vi "TestCloneAPI.vi"() -> ()   [LabVIEW 2014, in "SamplerModule.lvlib"]
uses:
  SamplerModule.lvlib
  SamplerPlugins/NISTSamplerPluginsBaseClass/TypeDefs/ConfigMeasurementParams.ctl
  SamplerPlugins/NISTSamplerPluginsBaseClass/TypeDefs/ConfigTriggerParams.ctl
  SamplerPlugins/NISTSamplerPluginsBaseClass/TypeDefs/ConfigACBandwidthParams.ctl
  SamplerPlugins/NISTSamplerPluginsBaseClass/TypeDefs/ConfigMultiPointParams.ctl
  SamplerPlugins/NISTSamplerPluginsBaseClass/TypeDefs/MultiPointReadingArrayParams.ctl
  SamplerPlugins/NISTSamplerPluginsBaseClass/TypeDefs/MultiPointReadingParams.ctl
  WfrmGenerator/WfrmPlugins/EventPluginBaseClass/TypeDefs/dblEvtSignalArray.ctl
  SamplerPlugins/NISTSamplerPluginsBaseClass/TypeDefs/CorrectionFactors.ctl
  <userlib>/NIST/ModuleAdminLib/ModuleAdmin/ModuleAdmin.lvclass
  PublicAPI/Arguments/Broadcasts/clDidInit.ctl
  <userlib>/NIST/ModuleAdminLib/ModuleAdmin/ModuleAdmin.lvclass/ModuleAdmin.ctl
  PublicAPI/Arguments/Requests/clStopArgument.ctl
  <userlib>/NIST/ModuleAdminLib/ModuleAdmin/Accessors/Read CloneRegRef.vi
  <userlib>/NIST/ModuleAdminLib/CloneRegistration/CloneRegistration.lvclass
  SamplerPlugins/NISTSamplerPluginsBaseClass/SamplerPluginsBase.lvclass
  SamplerPlugins/Simulation/Simulation.lvclass
  WfrmGenerator/WfrmPlugins/EventPluginBaseClass/BaseWfrmPlugin.lvclass
panel:
  in  "btnPref":bool
  in  "CorrectionFactors":T1
  in  "Plugin Type":u16(ring) items=["HP3458aDMM", "HIL Sampler", "NI Dyn3 Sampler", "NiPxi6123", "Sim"]
  in  "dblEventSignalArray":T2=array6x24000[144000 elements]
  in  "btnEvtSignal":bool
  in  "Loop Wait":u32=1000
  out "Waveform Chart":dbl[](graph)
  out "Stop":bool=TRUE
  out "Count":i32
  in  "btnLoopMultiPointReading":bool
  out "ReadingArray":dbl[](array[numeric])
  in  "btnInitiateMultiPoint":bool
  out "Waveform Graph":dbl[][](graph)
  out "MultiPointReadingArray":T3 {"Timestamp" format="%.6f"}
  in  "btnRequestMultiPointReading":bool
  in  "btnFetchMultiPoint":bool
  in  "btnReadMultiPoint":bool
  in  "ConfigMultiPointParams":T5={"iTriggerCount"=1, "iSampleCount"=4800, "eSampleClock"=2, "dSampleInterval"=0.00020833333333333332} {"eSampleClock" items=["NULL"=0, "Immediate"=1, "External"=2, "Software Trigger"=3, "Interval"=10]}
  in  "btnConfigMultiPoint":bool
  in  "eMeasCompleteDest":u16(ring) items=["None"=0, "External"=2]
  in  "btnConfigMeasCompDest":bool
  out "IsOverRange?":bool
  in  "dFrequencyVoltageRange":dbl
  in  "ConfigACBandwidthParams":T6
  in  "btnIsOverRange":bool
  in  "btnConfigACBandwidth":bool
  in  "btnConfigFreqVoltRange":bool
  in  "ConfigTriggerParams":T7={"eTriggerSource"=2, "dTriggerDelay"=0.0} {"eTriggerSource" items=["NULL", "Immediate", "External", "Software Trigger"]}
  in  "btnConfigTrigger":bool
  in  "btnInitiate":bool
  in  "iMaxTimeMillisecondsFetch":i32
  in  "btnFetch":bool
  in  "btnAbort":bool
  in  "btnReset":bool
  in  "btnInitializeDevice":bool
  in  "btnRequestReading":bool
  in  "iMaxTimeMilliseconds":i32
  in  "btnRead":bool
  in  "btnConfigMeasurement":bool
  in  "ConfigMeasurement":T8={"eFunction"=1, "dRange"=10.0, "dResolution"=0.0} {"eFunction" items=["NULL"=0, "DC Volts"=1, "AC Volts"=2, "DC Current"=3, "AC Current"=4, "Frequency"=104, "Period"=105, "AC Plus DC Volts"=106, "AC Plus DC Current"=107, "AC Coupled Direct Sampling"=1005, "DC Coupled Direct Sampling"=1006, "AC Coupled Sub Sampling"=1007, "DC Coupled Sub Sampling"=1008]}
  in  "btnLoadPlugin":bool
  out "Path":path
  in  "btnRequestINIPath":bool
  in  "btnRemove":bool
  out "Status Log":string
  out "Active Modules (Array)":string[](array[string])
  in  "btnAdd":bool
  in  "btnStop":bool
  in  "Select Module":i32(ring)=-1 caption="Select Module to send Request" items=["All"=-1]
  # "READING FROM .INI ONLY"
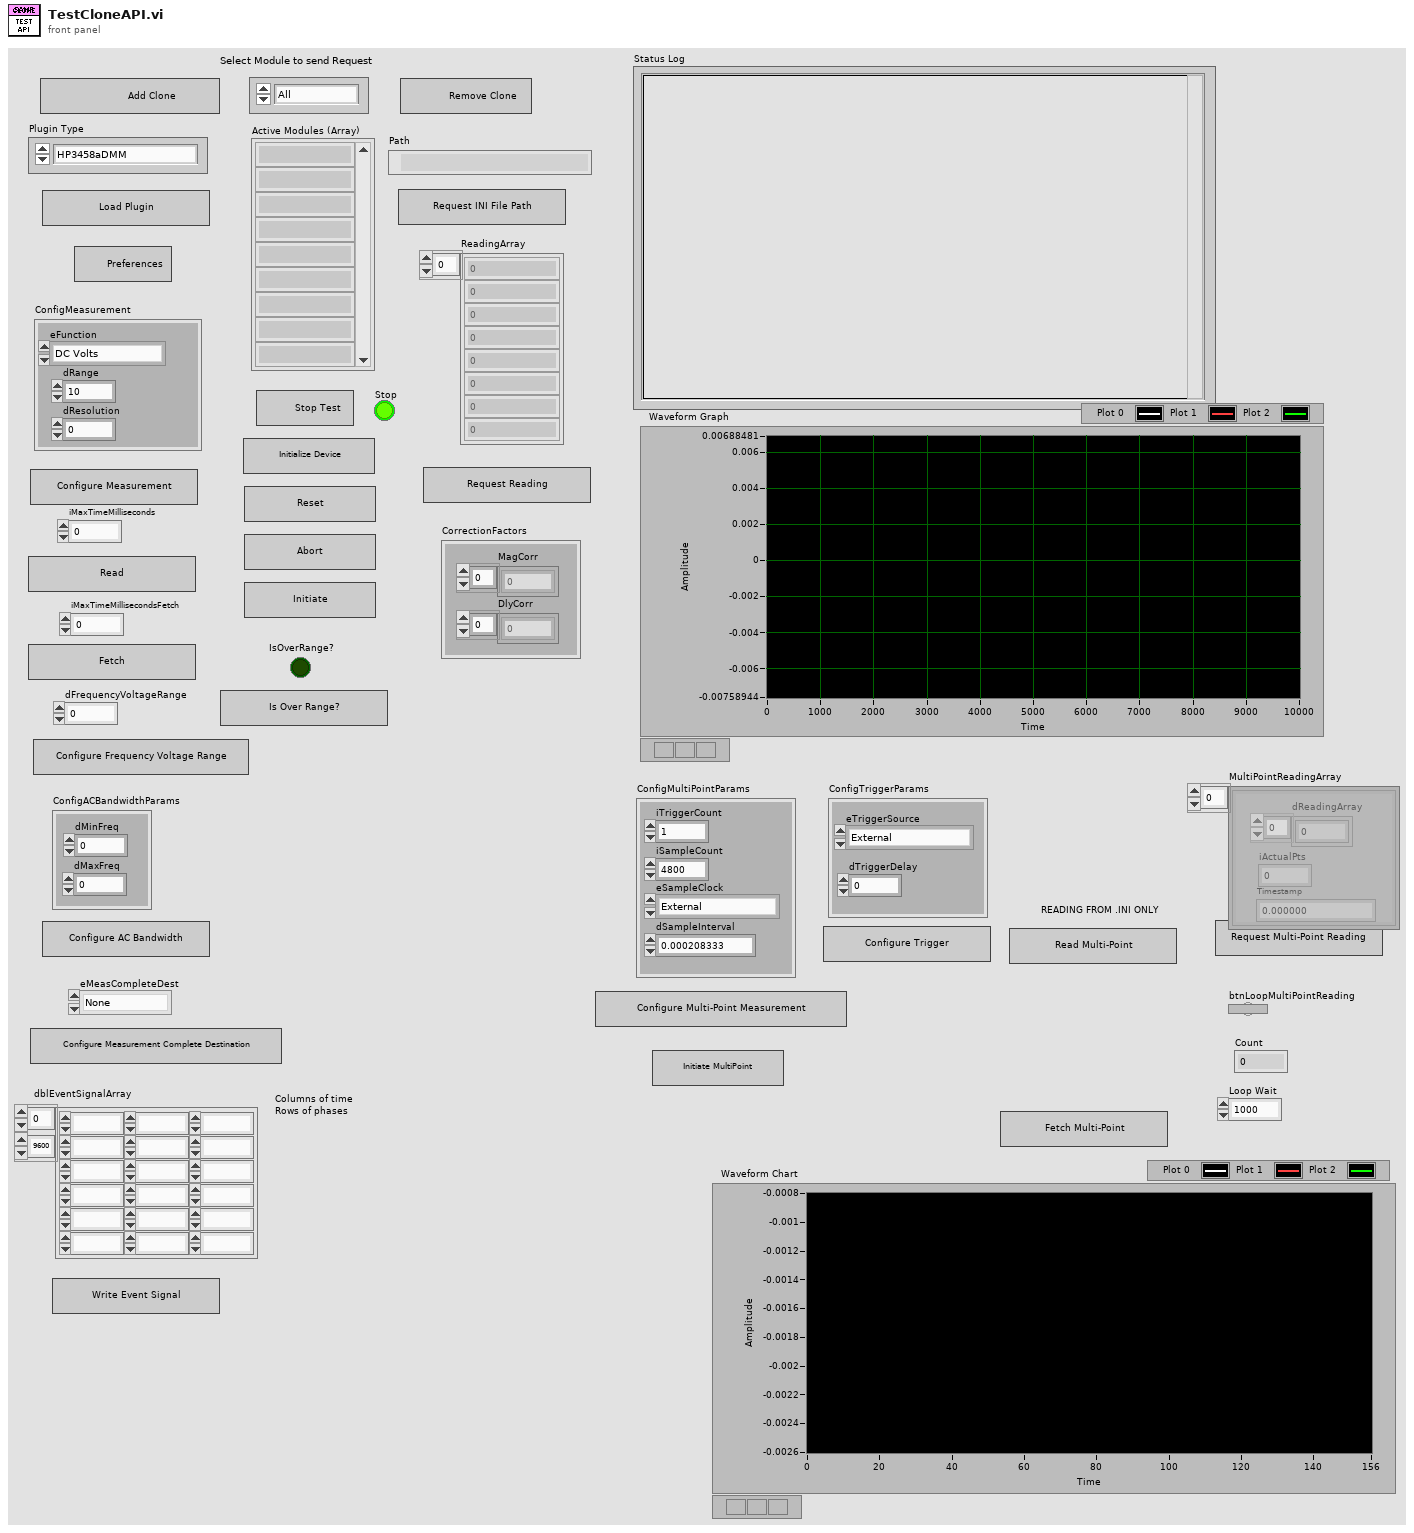
[diagram p1: front panel]
types:
  T1 = typedef "SamplerPlugins.lvlib/SamplerPluginsBase.lvclass/CorrectionFactors.ctl" = cluster{"MagCorr":dbl[], "DlyCorr":dbl[]}
  T2 = typedef "WfrmPlugins.lvlib/BaseWfrmPlugin.lvclass/dblEvtSignalArray.ctl" = dbl[][]
  T3 = typedef "SamplerPlugins.lvlib/SamplerPluginsBase.lvclass/MultiPointReadingArrayParams.ctl" = T4[]
  T4 = typedef "SamplerPlugins.lvlib/SamplerPluginsBase.lvclass/MultiPointReadingParams.ctl" = cluster{"dReadingArray":dbl[], "iActualPts":i32, "Timestamp":dbl}
  T5 = typedef "SamplerPlugins.lvlib/SamplerPluginsBase.lvclass/ConfigMultiPointParams.ctl" = cluster{"iTriggerCount":i32, "iSampleCount":i32, "eSampleClock":u16, "dSampleInterval":dbl}
  T6 = typedef "SamplerPlugins.lvlib/SamplerPluginsBase.lvclass/ConfigACBandwidthParams.ctl" = cluster{"dMinFreq":dbl, "dMaxFreq":dbl}
  T7 = typedef "SamplerPlugins.lvlib/SamplerPluginsBase.lvclass/ConfigTriggerParams.ctl" = cluster{"eTriggerSource":u16, "dTriggerDelay":dbl}
  T8 = typedef "SamplerPlugins.lvlib/SamplerPluginsBase.lvclass/ConfigMeasurementParams.ctl" = cluster{"eFunction":u16, "dRange":dbl, "dResolution":dbl}
  T9 = typedef "SamplerModule.lvlib/clBroadcastEvents.ctl" = cluster{"DidInit":refnum<user-event>, "StatusUpdate":refnum<user-event>, "ErrorReport":refnum<user-event>, "DidStop":refnum<user-event>, "PathToINI":refnum<user-event>, "GetReading":refnum<user-event>, "IsOverRange":refnum<user-event>, "GetMultiPointReading":refnum<user-event>, "MultiPointParams":refnum<user-event>, "MultiPointConfig":refnum<user-event>, "CorrFactors":refnum<user-event>}
  T10 = typedef "SamplerModule.lvlib/clDidInit.ctl" = cluster{"Init?":bool, "ModuleAdmin":refnum<class "ModuleAdmin.lvclass">}
  T11 = typedef "SamplerModule.lvlib/clStopArgument.ctl" = cluster{"Exit via Stop Module Req?":bool, "Wait for Module to stop?":bool, "ModuleAdmin":refnum<class "ModuleAdmin.lvclass">}
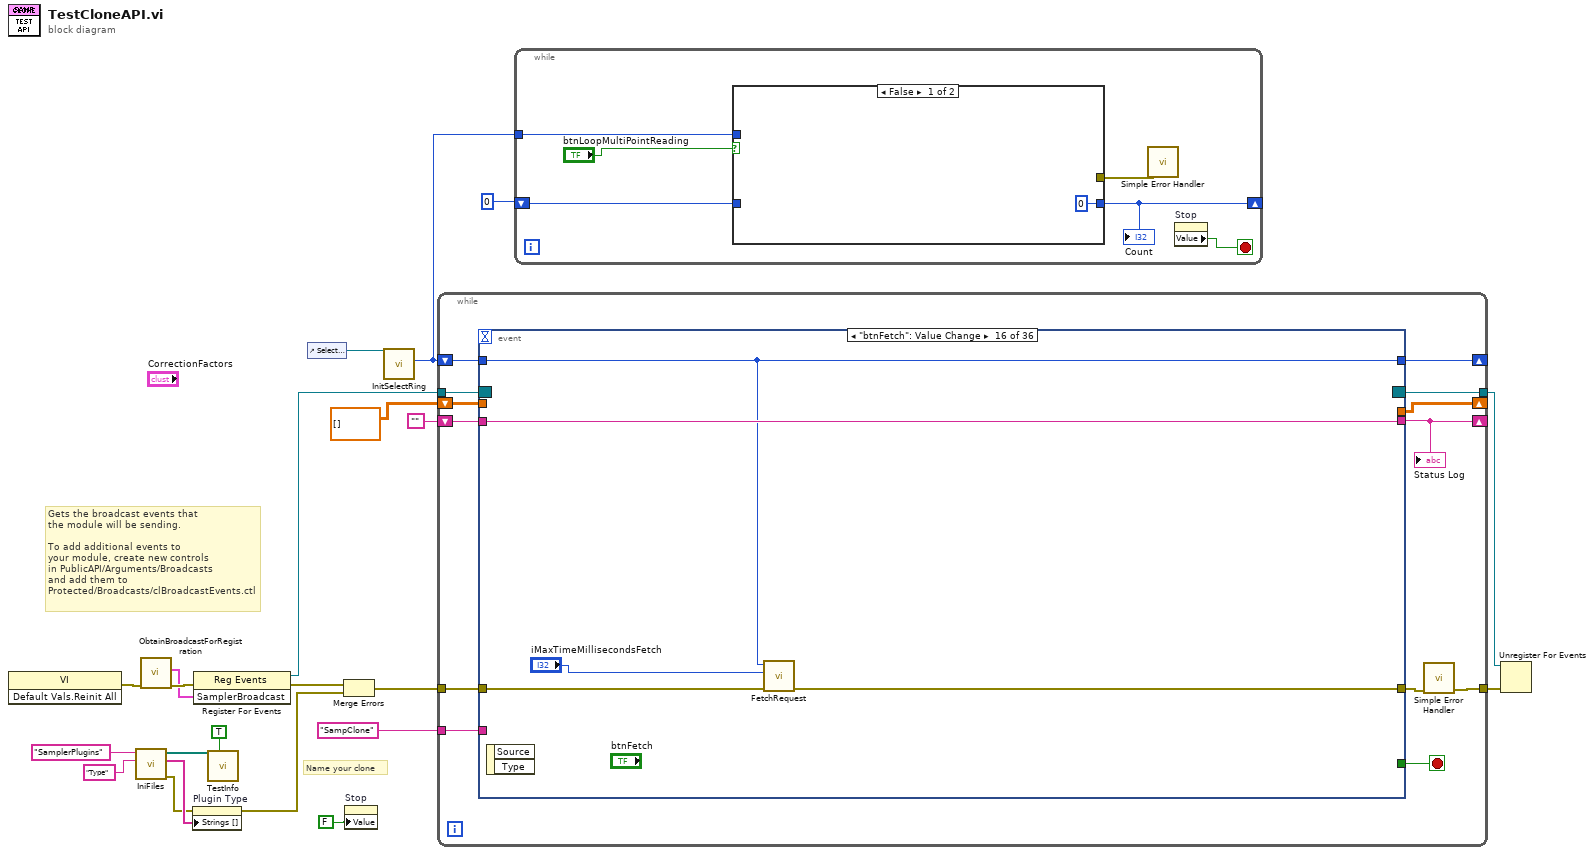
[diagram p0: block diagram]
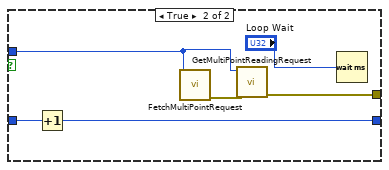
[diagram p2: hidden frame]
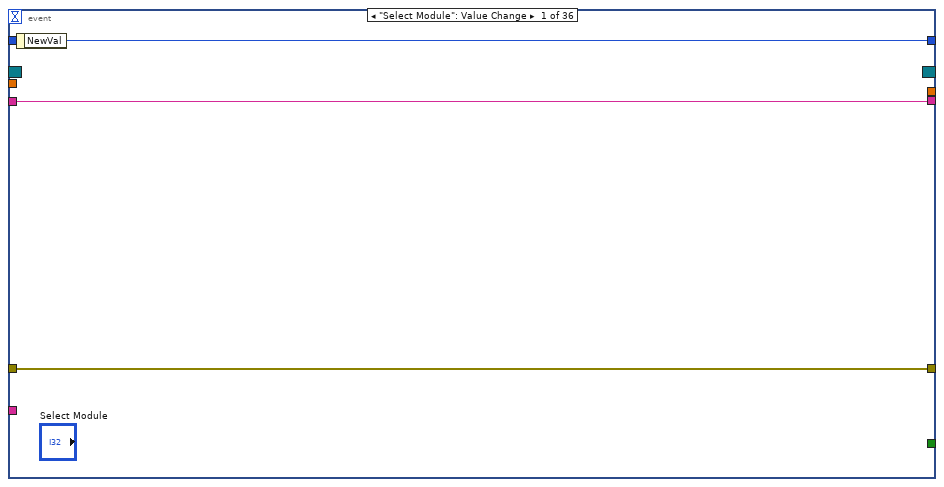
[diagram p3: hidden frame]
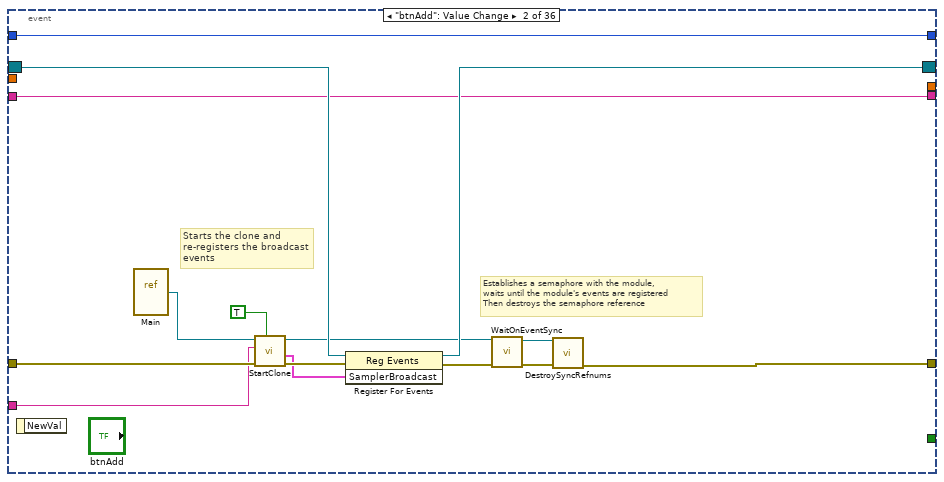
[diagram p4: hidden frame]
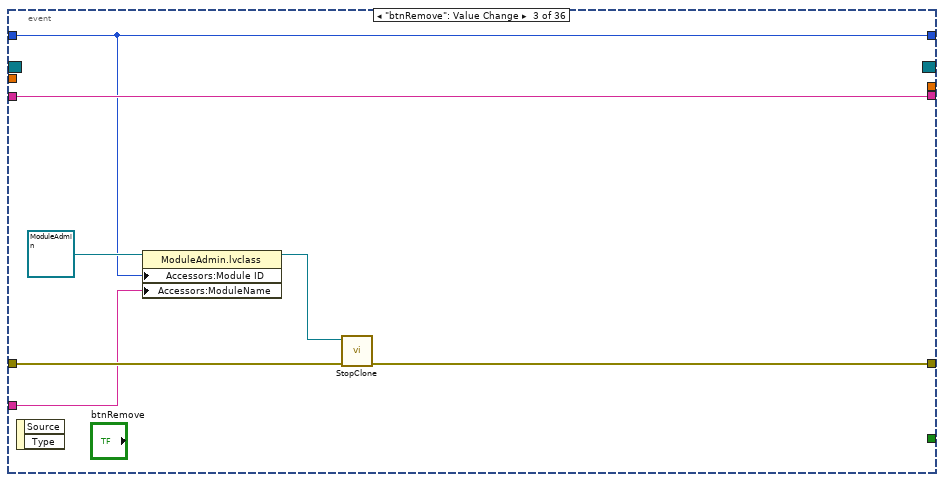
[diagram p5: hidden frame]
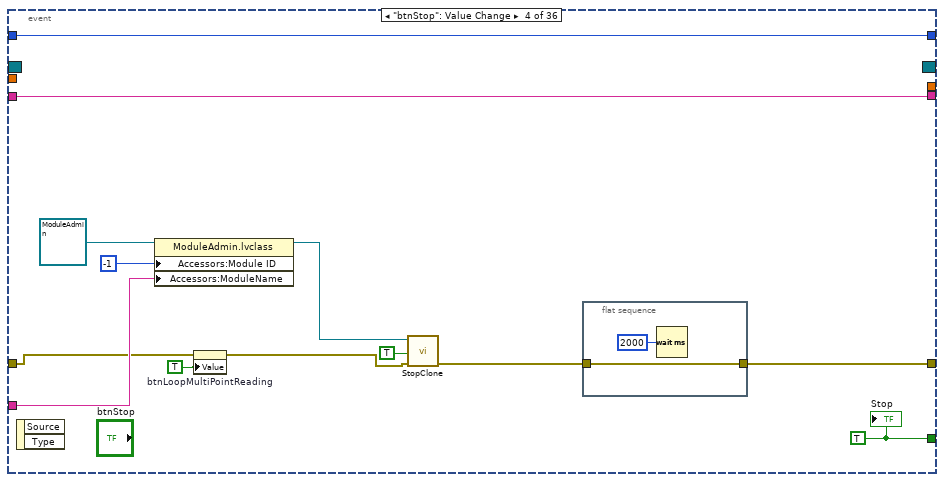
[diagram p6: hidden frame]
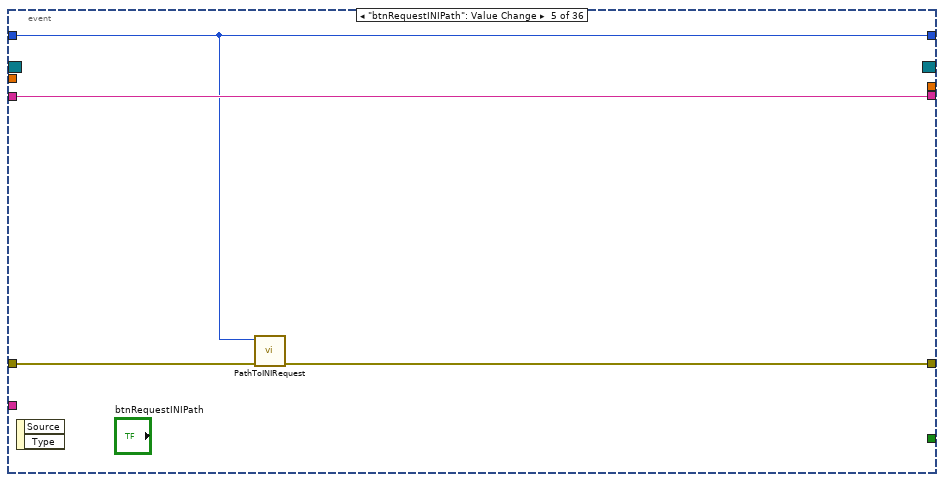
[diagram p7: hidden frame]
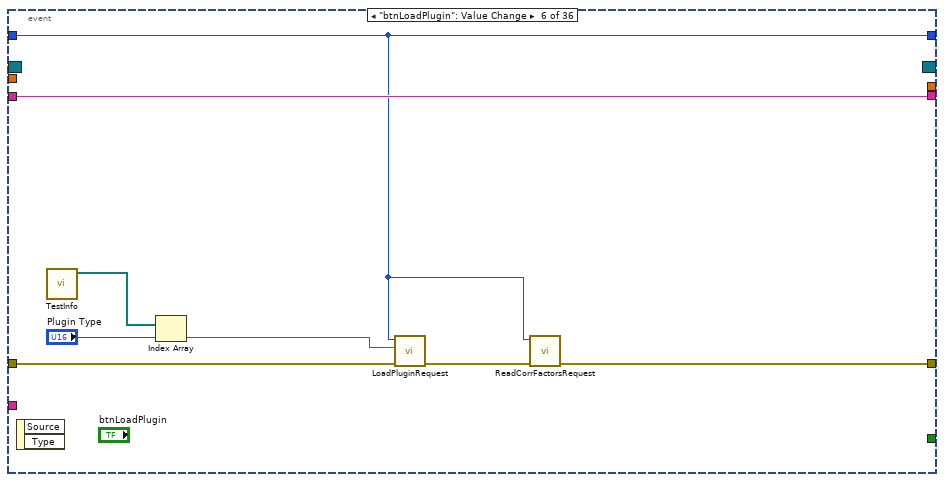
[diagram p8: hidden frame]
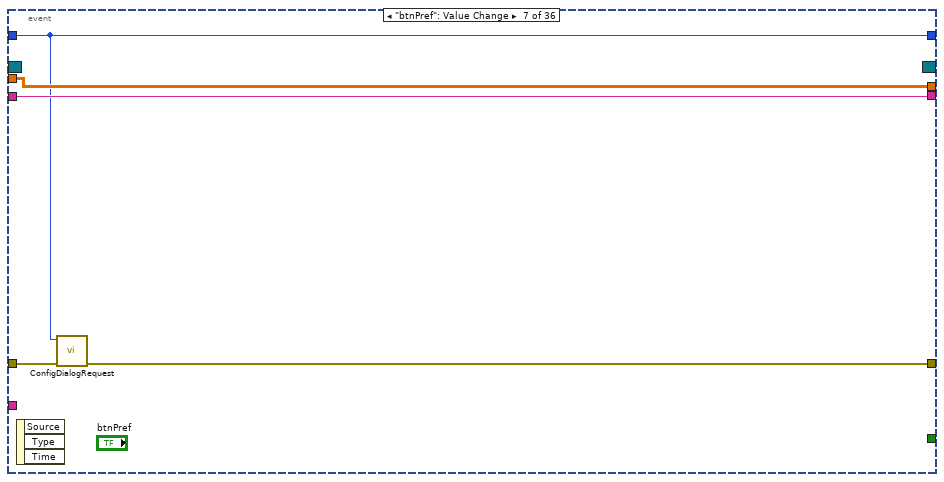
[diagram p9: hidden frame]
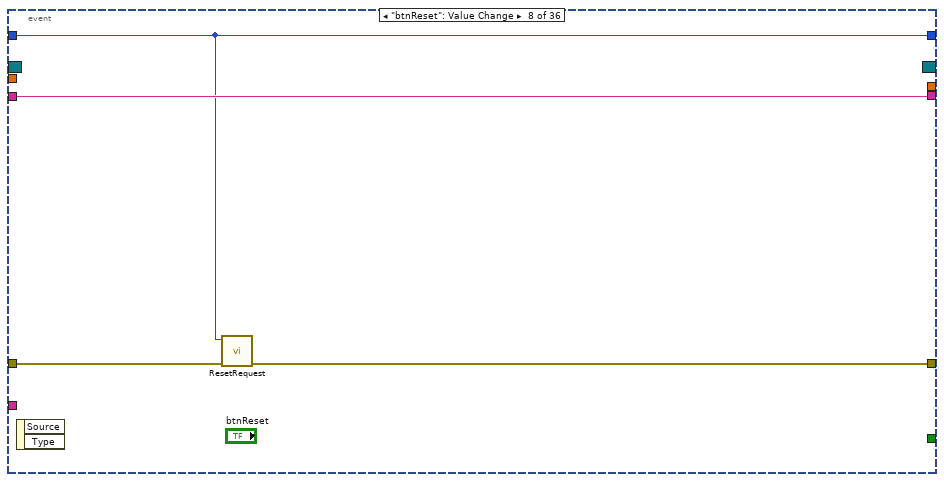
[diagram p10: hidden frame]
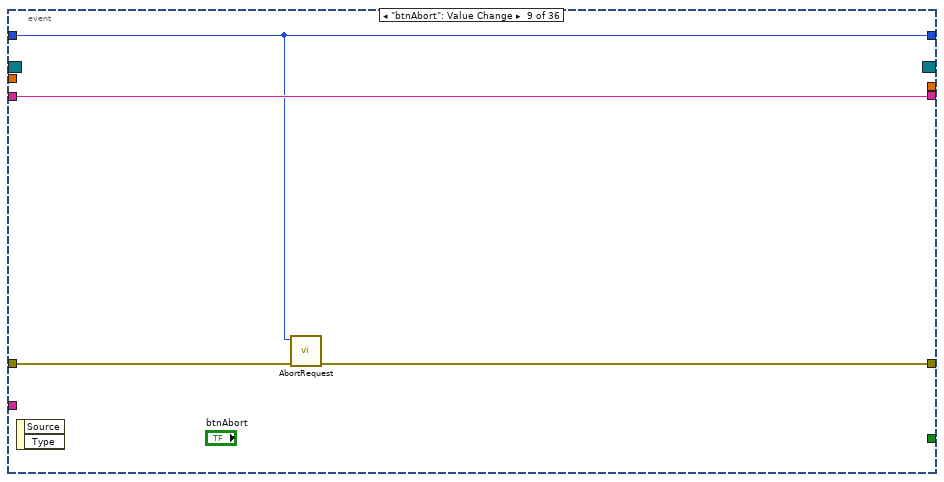
[diagram p11: hidden frame]
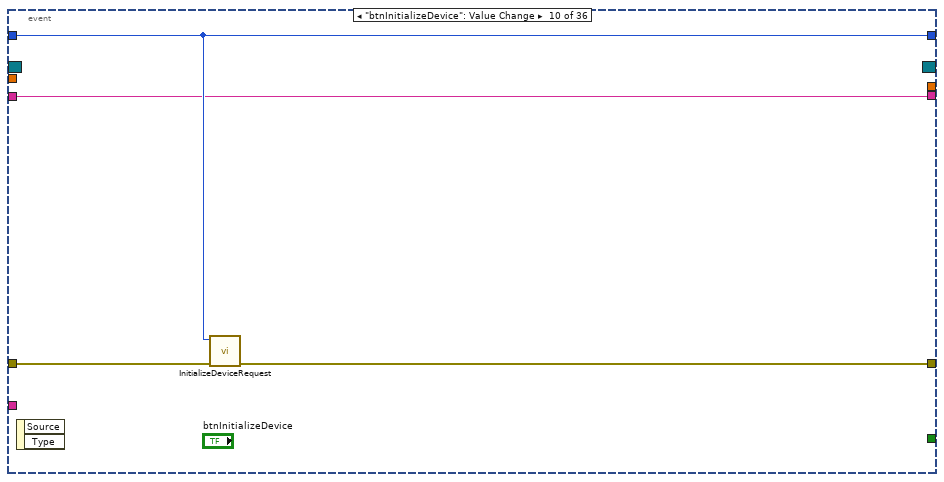
[diagram p12: hidden frame]
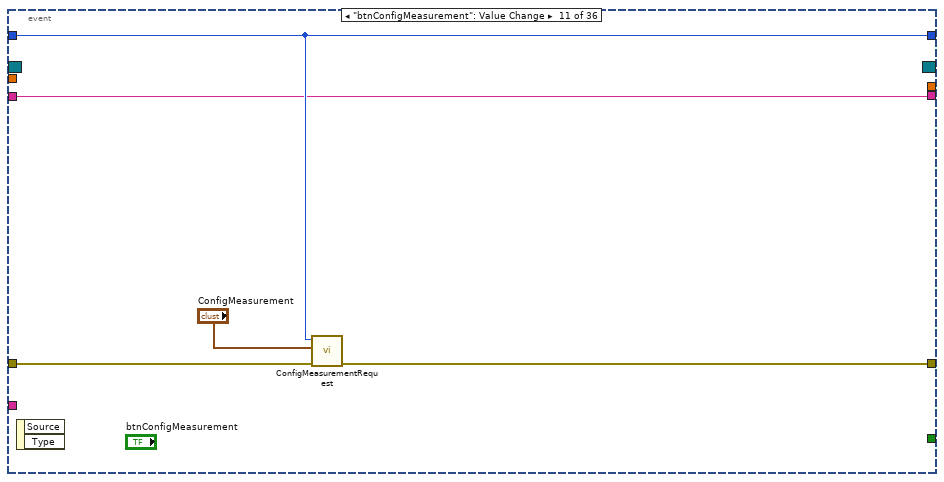
[diagram p13: hidden frame]
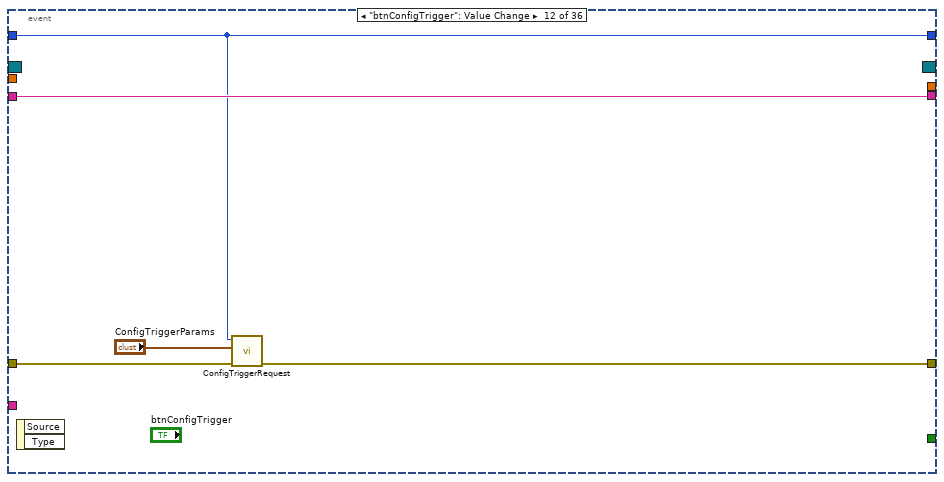
[diagram p14: hidden frame]
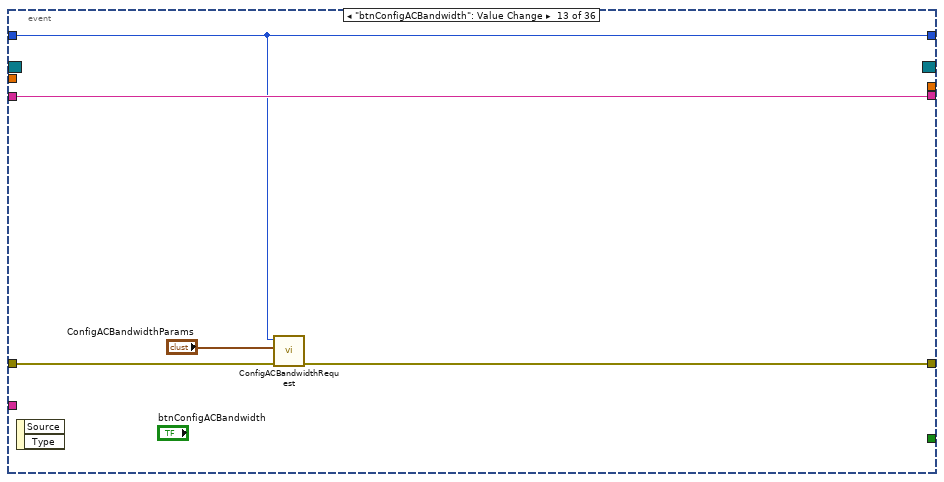
[diagram p15: hidden frame]
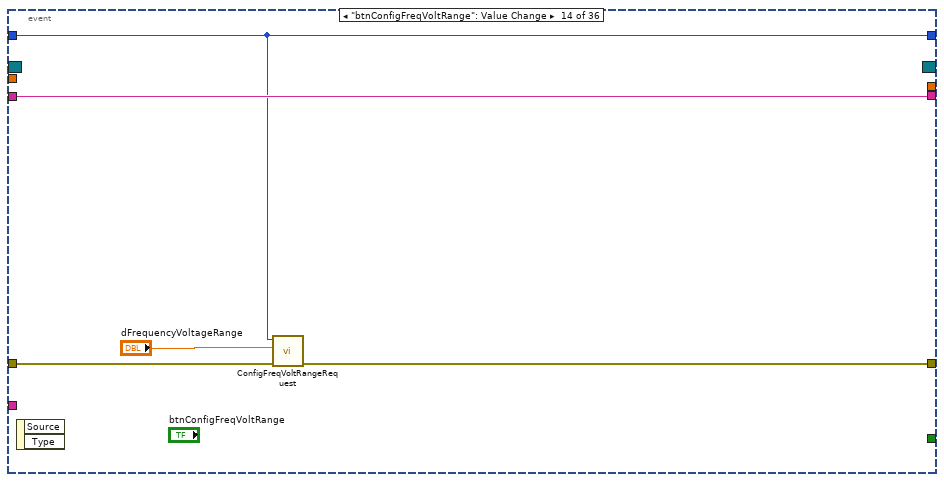
[diagram p16: hidden frame]
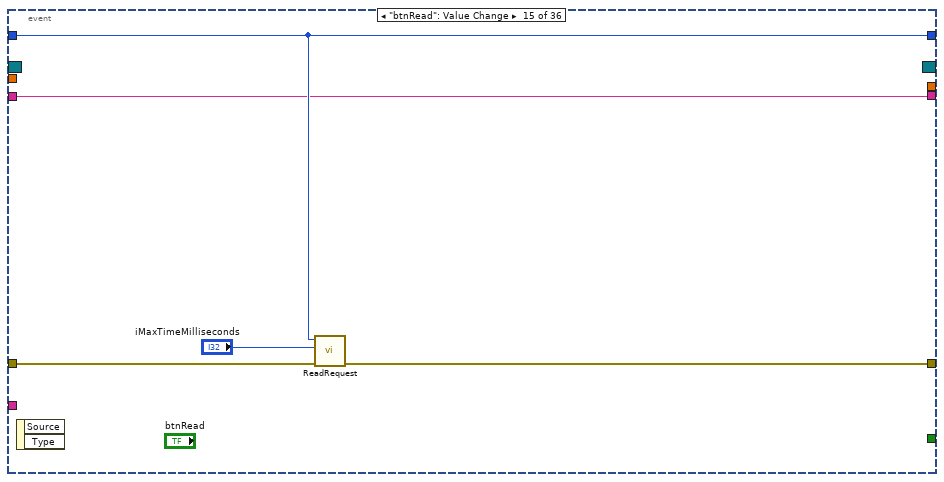
[diagram p17: hidden frame]
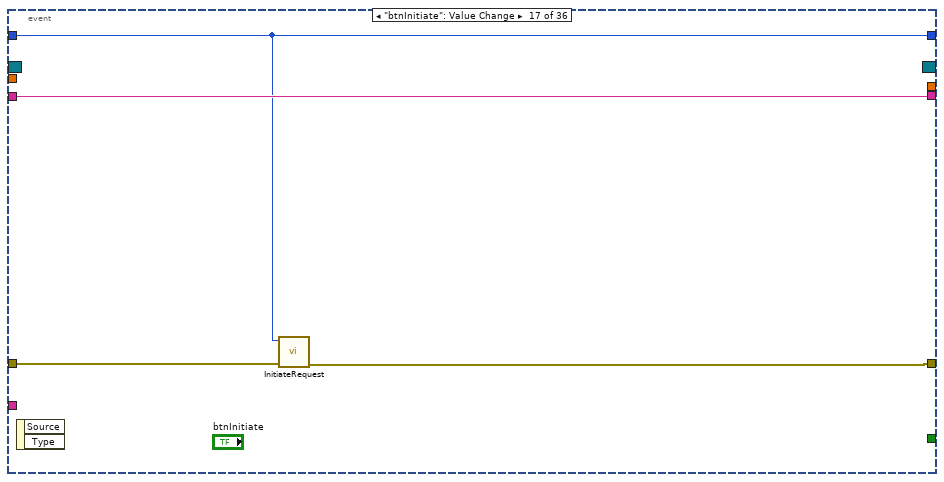
[diagram p18: hidden frame]
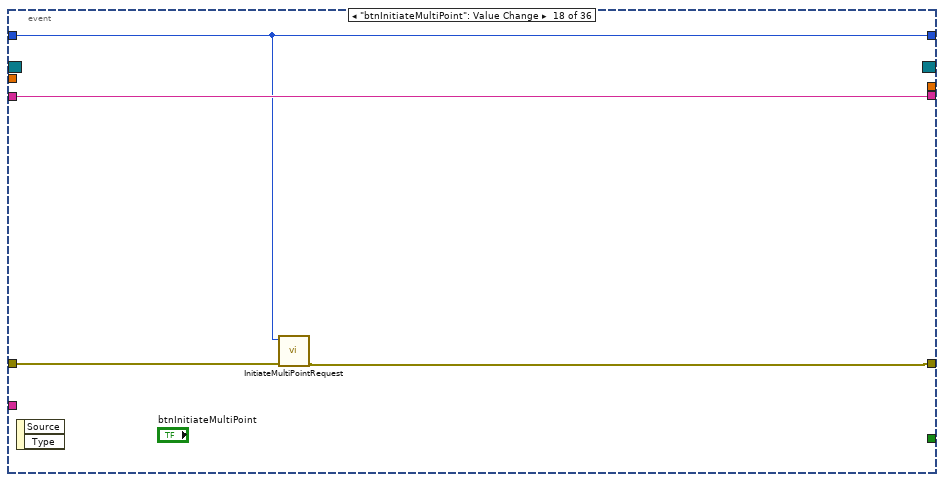
[diagram p19: hidden frame]
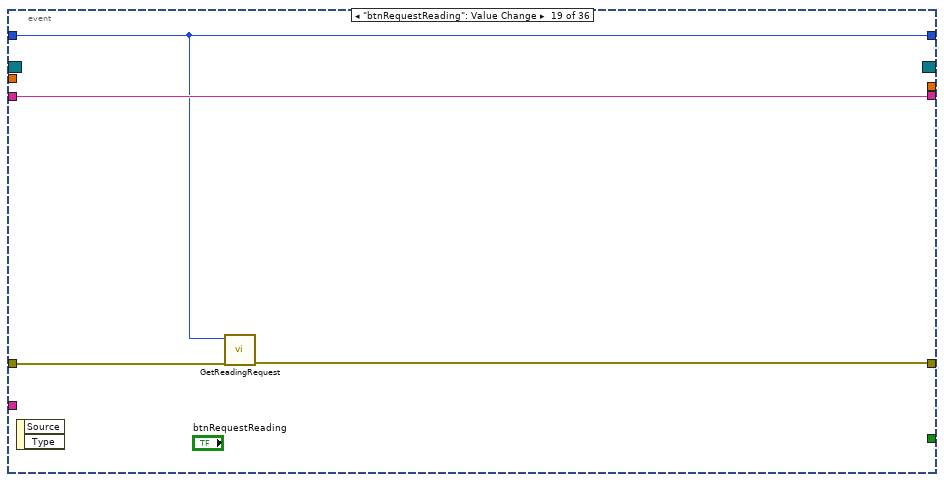
[diagram p20: hidden frame]
diagram:
  # "Name your clone"
  # "Gets the broadcast events that\nthe module will be sending.\n\nTo add additional events to\nyour module, create new controls\nin PublicAPI/Arguments/Broadcasts\nand add them to\nProtected/Broadcasts/clBroadcastEvents.ctl"
  n1 = invoke class="VI" method="Default Vals.Reinit All"() -> (error out=w21:errorcluster)  [unwired: 3 in, 2 out]
  n2 = call "IniFiles.vi"("iniKey"="Type", "name or relative path"="SamplerPlugins") -> ("error out"=w7:errorcluster, "Types"=w8:string[], "IniFilePaths"=w3:path[])  [unwired: 7 in]
  n3 = call "ObtainBroadcastForRegistration.vi"("error in (no error)"=w21) -> ("error out"=w20:errorcluster, "SamplerBroadcast"=w19:T9)  [unwired: 9 in]
  n4 = property on="Plugin Type" class="Ring (strict)"(error in=w7, "Strings []"=w8) -> (error out=w5:errorcluster)  [unwired: 1 in, 1 out]
  n5 = register-events(error in=w20, w19) -> (reference out=w17:refnum<event-registration>, error out=w18:errorcluster)  [unwired: 1 in]
  n6 = call "TestInfo.vi"("Set (f)"=TRUE, "PluginIniFilePaths"=w3) -> ()  [unwired: 9 in, 1 out]
  n7 = control-ref of="Select Module"() -> (w22:refnum<vi>)
  n8 = Merge Errors(w18, w5) -> (w6:errorcluster)
  n9 = property on="Stop" class="Bool (strict)"("Value"=FALSE ("Stop")) -> ()  [unwired: 2 in, 2 out]
  n10 = call "InitSelectRing.vi"("Ring Refnum"=w22) -> ("Module Ring Value"=w14:i32)  [unwired: 9 in, 1 out]
  n11 = while {
    shift-right: [w35] -> _
    shift-left: w14 -> [w26]
    tunnel: w6 -> [w33]
    tunnel: w17 -> [w30]
    tunnel: [w31] -> w2
    shift-right: [w29] -> _
    shift-left: "" -> [w28]
    tunnel: "SampClone" ("ModuleName") -> [w27]
    shift-right: [w24] -> _
    shift-left: dbl[][] [] -> [w25]
    tunnel: [w23] -> w1
    stop <- w34 stop-if-true
    n12 = event shown="[15] \"btnFetch\": Value Change" {
      selector: w30 -> [_ w45 _ _ _ _ _ _ _ _ _ _ _ _ _ _ _ _ _ _ _ _ _ _ _ _ _ _ _ _ _ _ _ _ _ _]
      dyn-events: [_ w44 _ _ _ _ _ _ _ _ _ _ _ _ _ _ _ _ _ _ _ _ _ _ _ _ _ _ _ _ _ _ _ _ _ _] -> w23
      timeout: _ -> [_ _ _ _ _ _ _ _ _ _ _ _ _ _ _ _ _ _ _ _ _ _ _ _ _ _ _ _ _ _ _ _ _ _ _ _]
      tunnel: w26 -> [_ w53 w56 w73 w78 w80 w89 w93 w97 w103 w109 w111 w115 w121 w129 w131 w137 w141 w143 w147 w151 w156 w161 w165 w169 w174 _ _ w243 w247 w258 w265 w272 w292 w301 w306]
      tunnel: [w38 w53 w56 w73 w78 w80 w89 w93 w97 w103 w109 w111 w115 w121 w129 w131 w137 w141 w143 w147 w151 w156 w161 w165 w169 w174 w200 w215 w243 w247 w258 w265 w272 w292 w301 w306] -> w35
      tunnel: [_ _ _ w72 _ _ _ _ _ _ _ _ _ _ _ _ _ _ _ _ _ _ _ _ _ _ _ _ _ _ _ _ _ _ _ _] -> w34
      tunnel: w33 -> [w36 w52 w59 w64 w77 w86 w92 w95 w99 w104 w107 w113 w118 w122 w127 w133 w136 w140 w145 w149 w155 w160 w164 w168 w172 w176 w205 w224 w240 w251 w254 w263 w270 w278 w299 w307]
      tunnel: [w36 w46 w58 w61 w76 w81 w88 w94 w98 w101 w106 w112 w117 w123 w126 w132 w135 w139 w144 w148 w154 w159 w163 w167 w171 w175 w189 w212 w234 w250 w253 w262 w269 w290 w294 w303] -> w32
      tunnel: [w37 w42 w60 w70 w79 w87 w91 w96 w100 w102 w105 w114 w119 w124 w125 w134 w138 w142 w146 w150 w152 w157 w162 w166 w170 w173 w193 w221 w237 w246 w259 w266 w273 w293 w300 w305] -> w29
      tunnel: w28 -> [w37 w42 w60 w70 w79 w87 w91 w96 w100 w102 w105 w114 w119 w124 w125 w134 w138 w142 w146 w150 w152 w157 w162 w166 w170 w173 w192 w222 w242 w246 w259 w266 w273 w293 w300 w305]
      tunnel: w27 -> [_ w41 w55 w67 _ _ _ _ _ _ _ _ _ _ _ _ _ _ _ _ _ _ _ _ _ _ _ _ _ _ _ _ _ _ _ _]
      tunnel: [_ _ _ _ _ _ w90 _ _ _ _ _ _ _ _ _ _ _ _ _ _ _ _ _ _ _ _ _ _ _ _ _ _ w275 _ w304] -> w24
      tunnel: w25 -> [_ _ _ _ _ _ w90 _ _ _ _ _ _ _ _ _ _ _ _ _ _ _ _ _ _ _ _ _ _ _ _ _ _ w276 _ w304]
      event "Select Module": Value Change {
        n13 = event-data() -> ("NewVal"=w38:i32)  [unwired: 1 in]
      }
      event "btnAdd": Value Change {
        # "Establishes a semaphore with the module,\nwaits until the module's events are registered\nThen destroys the semaphore reference"
        # "Starts the clone and\nre-registers the broadcast \nevents"
        n14 = event-data() -> ()  [unwired: 1 in, 1 out]
        n15 = vi-ref "Main.vi"() -> (w43:refnum<vi>)
        n16 = call "StartClone.vi"("ShowPanel? (F)"=TRUE, "error in (no error)"=w52, "ModuleName"=w41, "VI Refnum"=w43) -> ("error out"=w51:errorcluster, "SamplerBroadcastEvents"=w47:T9, "ModuleAdmin"=w40:refnum<class "ModuleAdmin.lvclass">)  [unwired: 5 in]
        n17 = register-events(reference=w45, error in=w51, w47) -> (reference out=w44:refnum<event-registration>, error out=w50:errorcluster)
        n18 = call <userlib>:"WaitOnEventSync.vi"("error in (no error)"=w50, "ModuleAdmin"=w40) -> ("error out"=w49:errorcluster, "ModuleAdmin"=w48:refnum<class "ModuleAdmin.lvclass">)  [unwired: 8 in]
        n19 = call <userlib>:"DestroySyncRefnums.vi"("error in (no error)"=w49, "ModuleAdmin"=w48) -> ("error out"=w46:errorcluster)  [unwired: 9 in]
      }
      event "btnRemove": Value Change {
        n20 = event-data() -> ()  [unwired: 1 in, 2 out]
        n21 = property class="ModuleAdmin.lvclass"(reference=refnum<class "ModuleAdmin.lvclass"> refnum ("ModuleAdmin.lvlib:ModuleAdmin.lvclass"), "Accessors:Module ID"=w56, "Accessors:ModuleName"=w55) -> (reference out=w54:refnum<class "ModuleAdmin.lvclass">)  [unwired: 1 in, 1 out]
        n22 = call "StopClone.vi"("error in (no error)"=w59, "ModuleAdmin"=w54) -> ("error out"=w58:errorcluster)  [unwired: 9 in]
      }
      event "btnStop": Value Change {
        w72 = TRUE
        n23 = event-data() -> ()  [unwired: 1 in, 2 out]
        n24 = property class="ModuleAdmin.lvclass"(reference=refnum<class "ModuleAdmin.lvclass"> refnum ("ModuleAdmin.lvlib:ModuleAdmin.lvclass"), "Accessors:Module ID"=-1 ("Module ID"), "Accessors:ModuleName"=w67) -> (reference out=w66:refnum<class "ModuleAdmin.lvclass">)  [unwired: 1 in, 1 out]
        n25 = property on="btnLoopMultiPointReading" class="Bool (strict)"(error in=w64, "Value"=TRUE ("btnLoopMultiPointReading")) -> (error out=w63:errorcluster)  [unwired: 1 in, 1 out]
        n26 = call "StopClone.vi"("error in (no error)"=w63, "Wait for Module to stop?"=TRUE, "ModuleAdmin"=w66) -> ("error out"=w62:errorcluster)  [unwired: 8 in]
        n27 = flat-sequence {
          tunnel: w62 -> [w74]
          tunnel: [w74] -> w61
          frame #0 {
            n28 = Wait (ms)(milliseconds to wait=u32 2000) -> ()  [unwired: 1 out]
          }
        }
        "Stop" <- w72
      }
      event "btnRequestINIPath": Value Change {
        n29 = event-data() -> ()  [unwired: 1 in, 2 out]
        n30 = call "PathToINIRequest.vi"("error in (no error)"=w77, "ModuleID"=w78) -> ("error out"=w76:errorcluster)  [unwired: 9 in]
      }
      event "btnLoadPlugin": Value Change {
        n31 = event-data() -> ()  [unwired: 1 in, 2 out]
        n32 = call "TestInfo.vi"() -> ("PluginIniFilePaths"=w85:path[])  [unwired: 11 in]
        n33 = Index Array(array=w85, index="Plugin Type") -> (element=w83:path)
        n34 = call "LoadPluginRequest.vi"("error in (no error)"=w86, "PathToPluginINI"=w83, "ModuleID"=w80) -> ("error out"=w82:errorcluster)  [unwired: 8 in]
        n35 = call "ReadCorrFactorsRequest.vi"("error in (no error)"=w82, "ModuleID"=w80) -> ("error out"=w81:errorcluster)  [unwired: 9 in]
      }
      event "btnPref": Value Change {
        n36 = event-data() -> ()  [unwired: 1 in, 3 out]
        n37 = call "ConfigDialogRequest.vi"("error in (no error)"=w92, "ModuleID"=w89) -> ("error out"=w88:errorcluster)  [unwired: 9 in]
      }
      event "btnReset": Value Change {
        n38 = event-data() -> ()  [unwired: 1 in, 2 out]
        n39 = call "ResetRequest.vi"("error in (no error)"=w95, "ModuleID"=w93) -> ("error out"=w94:errorcluster)  [unwired: 9 in]
      }
      event "btnAbort": Value Change {
        n40 = event-data() -> ()  [unwired: 1 in, 2 out]
        n41 = call "AbortRequest.vi"("error in (no error)"=w99, "ModuleID"=w97) -> ("error out"=w98:errorcluster)  [unwired: 9 in]
      }
      event "btnInitializeDevice": Value Change {
        n42 = event-data() -> ()  [unwired: 1 in, 2 out]
        n43 = call "InitializeDeviceRequest.vi"("error in (no error)"=w104, "ModuleID"=w103) -> ("error out"=w101:errorcluster)  [unwired: 9 in]
      }
      event "btnConfigMeasurement": Value Change {
        n44 = event-data() -> ()  [unwired: 1 in, 2 out]
        n45 = call "ConfigMeasurementRequest.vi"("error in (no error)"=w107, "ConfigMeasurement"="ConfigMeasurement", "ModuleID"=w109) -> ("error out"=w106:errorcluster)  [unwired: 8 in]
      }
      event "btnConfigTrigger": Value Change {
        n46 = event-data() -> ()  [unwired: 1 in, 2 out]
        n47 = call "ConfigTriggerRequest.vi"("error in (no error)"=w113, "ConfigTriggerParams"="ConfigTriggerParams", "ModuleID"=w111) -> ("error out"=w112:errorcluster)  [unwired: 8 in]
      }
      event "btnConfigACBandwidth": Value Change {
        n48 = event-data() -> ()  [unwired: 1 in, 2 out]
        n49 = call "ConfigACBandwidthRequest.vi"("error in (no error)"=w118, "ConfigACBandwidthParams"="ConfigACBandwidthParams", "ModuleID"=w115) -> ("error out"=w117:errorcluster)  [unwired: 8 in]
      }
      event "btnConfigFreqVoltRange": Value Change {
        n50 = event-data() -> ()  [unwired: 1 in, 2 out]
        n51 = call "ConfigFreqVoltRangeRequest.vi"("error in (no error)"=w122, "dFrequencyVoltageRange"="dFrequencyVoltageRange", "ModuleID"=w121) -> ("error out"=w123:errorcluster)  [unwired: 8 in]
      }
      event "btnRead": Value Change {
        n52 = event-data() -> ()  [unwired: 1 in, 2 out]
        n53 = call "ReadRequest.vi"("error in (no error)"=w127, "iMaxTimeMilliseconds"="iMaxTimeMilliseconds", "ModuleID"=w129) -> ("error out"=w126:errorcluster)  [unwired: 8 in]
      }
      event "btnFetch": Value Change {
        n54 = event-data() -> ()  [unwired: 1 in, 2 out]
        n55 = call "FetchRequest.vi"("error in (no error)"=w133, "iMaxTimeMilliseconds"="iMaxTimeMillisecondsFetch", "ModuleID"=w131) -> ("error out"=w132:errorcluster)  [unwired: 8 in]
      }
      event "btnInitiate": Value Change {
        n56 = event-data() -> ()  [unwired: 1 in, 2 out]
        n57 = call "InitiateRequest.vi"("error in (no error)"=w136, "ModuleID"=w137) -> ("error out"=w135:errorcluster)  [unwired: 9 in]
      }
      event "btnInitiateMultiPoint": Value Change {
        n58 = event-data() -> ()  [unwired: 1 in, 2 out]
        n59 = call "InitiateMultiPointRequest.vi"("error in (no error)"=w140, "ModuleID"=w141) -> ("error out"=w139:errorcluster)  [unwired: 9 in]
      }
      event "btnRequestReading": Value Change {
        n60 = event-data() -> ()  [unwired: 1 in, 2 out]
        n61 = call "GetReadingRequest.vi"("error in (no error)"=w145, "ModuleID"=w143) -> ("error out"=w144:errorcluster)  [unwired: 9 in]
      }
      event "btnIsOverRange": Value Change {
        n62 = event-data() -> ()  [unwired: 1 in, 2 out]
        n63 = call "IsOverRangeRequest.vi"("error in (no error)"=w149, "ModuleID"=w147) -> ("error out"=w148:errorcluster)  [unwired: 9 in]
      }
      event "btnConfigMeasCompDest": Value Change {
        n64 = event-data() -> ()  [unwired: 1 in, 2 out]
        n65 = call "ConfigMeasCompDestRequest.vi"("error in (no error)"=w155, "eMeasCompleteDest"="eMeasCompleteDest", "ModuleID"=w151) -> ("error out"=w154:errorcluster)  [unwired: 8 in]
      }
      event "btnConfigMultiPoint": Value Change {
        n66 = event-data() -> ()  [unwired: 1 in, 2 out]
        n67 = call "WriteMultiPointConfigRequest.vi"("error in (no error)"=w160, "MultiPointConfig"="ConfigMultiPointParams", "ModuleID"=w156) -> ("error out"=w159:errorcluster)  [unwired: 8 in]
      }
      event "btnReadMultiPoint": Value Change {
        n68 = event-data() -> ()  [unwired: 1 in, 2 out]
        n69 = call "ReadMultiPointRequest.vi"("error in (no error)"=w164, "ModuleID"=w161) -> ("error out"=w163:errorcluster)  [unwired: 9 in]
      }
      event "btnFetchMultiPoint": Value Change {
        n70 = event-data() -> ()  [unwired: 1 in, 2 out]
        n71 = call "FetchMultiPointRequest.vi"("error in (no error)"=w168, "ModuleID"=w165) -> ("error out"=w167:errorcluster)  [unwired: 9 in]
      }
      event "btnRequestMultiPointReading": Value Change {
        n72 = event-data() -> ()  [unwired: 1 in, 2 out]
        n73 = call "GetMultiPointReadingRequest.vi"("error in (no error)"=w172, "ModuleID"=w169) -> ("error out"=w171:errorcluster)  [unwired: 9 in]
      }
      event "btnLoopMultiPointReading": Value Change {
        n74 = event-data() -> ()  [unwired: 1 in, 2 out]
        n75 = disable-structure shown="Disabled" {
          disable-tunnel: w176 -> [w179 w182]
          disable-tunnel: [w178 w182] -> w175
          disable-tunnel: w174 -> [w177 _]
          frame Disabled {
            n76 = call "ReadMultiPointRequest.vi"("error in (no error)"=w179, "ModuleID"=w177) -> ("error out"=w181:errorcluster, 10:w180)  [unwired: 8 in]
            n77 = call "GetMultiPointReadingRequest.vi"("error in (no error)"=w181, "ModuleID"=w177) -> ("error out"=w178:errorcluster)  [unwired: 9 in]
          }
          frame Enabled {
          }
        }
      }
      event User Event {
        # "Adds the module ID to the \nSelect Module ring"
        # "Time stamp and add the DidInit message to the log"
        # "The data types for the broadcast messages\nare in PublicAPI/Broadcasts"
        n78 = event-data() -> ("Data"=w204:variant)  [unwired: 1 in]
        n79 = Variant To Data(error in=w205, type=T10 {"Init?"=FALSE, "ModuleAdmin"=refnum} ("clDidInit"), Variant=w204) -> (data=w197:T10, error out=w202:errorcluster)
        n80 = Unbundle By Name(w197) -> ("ModuleAdmin"=w187:refnum<class "ModuleAdmin.lvclass">)
        n81 = Get Date/Time In Seconds() -> (seconds since 1Jan1904=w195:timestamp)
        n82 = property class="ModuleAdmin.lvclass"(reference=w187) -> ("Accessors:ModuleName"=w185:string, "Accessors:Module ID"=w184:i32, "Accessors:CloneRegRef"=w183:refnum<data-value>)  [unwired: 1 in, 2 out]
        n83 = Get Date/Time String(date format (0)=enum16{"short", "long", "abbreviated"}."short", seconds (now)=w195, want seconds? (F)=TRUE) -> (time string=w198:string)  [unwired: 1 out]
        n84 = Format Into String(format string="%s: %s:%d %s \\r", initial string=w192, w198, w185, w184, "Did Init.") -> (resulting string=w193:string, error out=w190:errorcluster)  [unwired: 1 in]
        n85 = control-ref of="Select Module"() -> (w201:refnum<vi>)
        n86 = call "UpdateSelectRing.vi"("error in (no error)"=w202, "CloneRegRef"=w183, "Ring Refnum"=w201) -> ("error out"=w191:errorcluster, "ActiveModules"=→"Active Modules (Array)":string[], "Module Ring Value"=w200:i32)  [unwired: 6 in]
        n87 = Merge Errors(w191, w190) -> (w189:errorcluster)
      }
      event User Event {
        # "Time stamp and add the Stop message to the log"
        # "The Stop Argument  is found in\nPublicAPI/Arguments/Requests"
        n88 = event-data() -> ("Data"=w223:variant)  [unwired: 1 in]
        n89 = Variant To Data(error in=w224, type=T11 {"Exit via Stop Module Req?"=FALSE, "Wait for Module to stop?"=FALSE, "ModuleAdmin"=refnum} ("Stop Argument"), Variant=w223) -> (data=w219:T11, error out=w218:errorcluster)
        n90 = Unbundle By Name(w219) -> ("ModuleAdmin"=w210:refnum<class "ModuleAdmin.lvclass">)
        n91 = property class="ModuleAdmin.lvclass"(reference=w210) -> ("Accessors:ModuleName"=w208:string, "Accessors:Module ID"=w207:i32, "Accessors:CloneRegRef"=w206:refnum<data-value>)  [unwired: 1 in, 2 out]
        n92 = Get Date/Time In Seconds() -> (seconds since 1Jan1904=w226:timestamp)
        n93 = Get Date/Time String(date format (0)=enum16{"short", "long", "abbreviated"}."short", seconds (now)=w226, want seconds? (F)=TRUE) -> (time string=w228:string)  [unwired: 1 out]
        n94 = Format Into String(format string="%s: %s:%d %s \\r", initial string=w222, w228, w208, w207, "Stopping") -> (resulting string=w221:string, error out=w213:errorcluster)  [unwired: 1 in]
        n95 = control-ref of="Select Module"() -> (w217:refnum<vi>)
        n96 = call "UpdateSelectRing.vi"("error in (no error)"=w218, "CloneRegRef"=w206, "Ring Refnum"=w217) -> ("error out"=w214:errorcluster, "ActiveModules"=w216:string[], "Module Ring Value"=w215:i32)  [unwired: 6 in]
        n97 = local write "Active Modules (Array)"(w216) -> ()
        n98 = Merge Errors(w214, w213) -> (w212:errorcluster)
      }
      event User Event {
        # "Time stamp and add the Status message to the log"
        # "The data types for the broadcast messages\nare in PublicAPI/Broadcasts"
        n99 = event-data() -> ("Data"=w239:variant)  [unwired: 1 in]
        n100 = Variant To Data(error in=w240, type="", Variant=w239) -> (data=w229:string, error out=w236:errorcluster)
        n101 = Get Date/Time In Seconds() -> (seconds since 1Jan1904=w238:timestamp)
        n102 = Get Date/Time String(date format (0)=enum16{"short", "long", "abbreviated"}."short", seconds (now)=w238, want seconds? (F)=TRUE) -> (time string=w231:string)  [unwired: 1 out]
        n103 = Format Into String(format string="%s: %s \\r", initial string=w242, w231, w229) -> (resulting string=w237:string, error out=w235:errorcluster)  [unwired: 1 in]
        n104 = Merge Errors(w236, w235) -> (w234:errorcluster)
      }
      event User Event {
        # "#CodeNeeded\nThis is a very crude error handler\nA better error handler will be needed"
        n105 = event-data() -> ("ModuleID"=w249:i32, "Data"=w252:variant)  [unwired: 1 in]
        n106 = Variant To Data(error in=w251, type=errorcluster {"status"=FALSE, "code"=0, "source"=""} ("error constant"), Variant=w252) -> (data=w244:errorcluster, error out=w250:errorcluster)
        n107 = Number To Decimal String(number=w249) -> (decimal integer string=w248:string)  [unwired: 1 in]
        n108 = call <vilib>:"General Error Handler.vi"("[error source] (\" \")"=w248, "error in (no error)"=w244) -> ()  [unwired: 9 in, 5 out]
      }
      event User Event {
        n109 = event-data() -> ("Data"=w256:variant)  [unwired: 1 in, 1 out]
        n110 = Variant To Data(error in=w254, type=path "" ("Path"), Variant=w256) -> (data=→"Path":path, error out=w253:errorcluster)
      }
      event User Event {
        n111 = event-data() -> ("Data"=w264:variant)  [unwired: 1 in, 1 out]
        n112 = Variant To Data(error in=w263, type=dbl[] [], Variant=w264) -> (data=→"ReadingArray":dbl[], error out=w262:errorcluster)
      }
      event User Event {
        n113 = event-data() -> ("Data"=w271:variant)  [unwired: 1 in, 1 out]
        n114 = Variant To Data(error in=w270, type=FALSE ("IsOverRange?"), Variant=w271) -> (data=→"IsOverRange?":bool, error out=w269:errorcluster)
      }
      event User Event {
        n115 = event-data() -> ("Data"=w291:variant)  [unwired: 1 in, 1 out]
        n116 = invoke on="Waveform Graph" class="WFGraph (strict)" method="Reinit To Default"(error in=w278) -> (error out=w277:errorcluster)  [unwired: 2 in, 2 out]
        n117 = Variant To Data(error in=w277, type=T3 [] ("MultiPointReadingArray"), Variant=w291) -> (data=w287:T3, error out=w290:errorcluster)
        "MultiPointReadingArray" <- w287
        n118 = Index Array(array=w287, index=0) -> (element=w288:T4)
        n119 = Index Array(array=w287, index=1) -> (element=w282:T4)
        n120 = Index Array(array=w287, index=2) -> (element=w283:T4)
        n121 = Unbundle By Name(w288) -> ("dReadingArray"=w274:dbl[])
        "Waveform Chart" <- w274
        n122 = Unbundle By Name(w282) -> ("dReadingArray"=w281:dbl[])
        n123 = Unbundle By Name(w283) -> ("dReadingArray"=w280:dbl[])
        n124 = Build Array(w274, w281, w280) -> (→"Waveform Graph":dbl[][])
        n125 = Build Array (concatenate)(w276, w274) -> (w275:dbl[][])
      }
      event User Event {
        n126 = event-data() -> ("Data"=w298:variant)  [unwired: 1 in, 1 out]
        n127 = Variant To Data(error in=w299, type=T1 {"MagCorr"=[], "DlyCorr"=[]} ("CorrectionFactors"), Variant=w298) -> (data=w296:T1, error out=w295:errorcluster)
        n128 = property on="CorrectionFactors" class="Clust (strict)"(error in=w295, "Value"=w296) -> (error out=w294:errorcluster)  [unwired: 1 in, 1 out]
      }
      event "btnEvtSignal": Value Change {
        n129 = event-data() -> ()  [unwired: 1 in, 1 out]
        n130 = call "WriteEvtSignalRequest.vi"("error in (no error)"=w307, "EvtSignal"="dblEventSignalArray", "ModuleID"=w306) -> ("error out"=w303:errorcluster)  [unwired: 8 in]
      }
    }
    "Status Log" <- w29
    n131 = call <vilib>:"Simple Error Handler.vi"("error in (no error)"=w32) -> ("error out"=w31:errorcluster)  [unwired: 4 in, 4 out]
  }
  n132 = while {
    tunnel: w14 -> [w311]
    shift-right: [w308] -> _
    shift-left: 0 -> [w309]
    stop <- w310 stop-if-true
    n133 = case shown="False" "btnLoopMultiPointReading" {
      tunnel: w311 -> [_ w319]
      tunnel: [_ w318] -> w313
      tunnel: w309 -> [_ w317]
      tunnel: [0 w316] -> w308
      frame False {
      }
      frame True {
        n134 = Increment(x=w317) -> (x+1=w316:i32)
        n135 = call "FetchMultiPointRequest.vi"("ModuleID"=w319) -> ("error out"=w320:errorcluster)  [unwired: 10 in]
        n136 = call "GetMultiPointReadingRequest.vi"("error in (no error)"=w320, "ModuleID"=w319) -> ("error out"=w318:errorcluster)  [unwired: 9 in]
        n137 = Wait (ms)(milliseconds to wait="Loop Wait") -> ()  [unwired: 1 out]
      }
    }
    "Count" <- w308
    n138 = call <vilib>:"Simple Error Handler.vi"("error in (no error)"=w313) -> ()  [unwired: 4 in, 5 out]
    n139 = property on="Stop" class="Bool (strict)"() -> ("Value"=w310:bool)  [unwired: 2 in, 2 out]
  }
  n140 = Unregister For Events(event registration refnum=w1, error in=w2) -> ()  [unwired: 1 out]
